vi "Test Status Correct When Collecting Case Result.vi"(8 "error in (no error)":errorcluster, 11 "Test Case In":refnum<class "Result Collector Tests.lvclass">) -> (0 "error out":errorcluster, 3 "Test Case Out":refnum<class "Result Collector Tests.lvclass">)   [LabVIEW 2020, in "Result Collector Tests.lvclass"]
uses:
  Result Collector Tests.lvclass
  C:/Program Files (x86)/National Instruments/LabVIEW 2020/vi.lib/Astemes/LUnit/Test Case.lvclass
  source/Framework/Result Collector/Result Collector.lvclass
  source/Rewrite Project/Result/Result.ctl
  source/Rewrite Project/Result/Status.ctl
  source/Rewrite Project/Result/Type.ctl
  source/Framework/Result Collector/Result Collector.lvclass/Result Collector.ctl
  <vilib>/Astemes/LUnit/Test Case.lvclass/Test Case.ctl
  7d523b10-b8d1-4baa-9334-5865d033fd32.vi
  source/Framework/Result Collector/Public/API/Collect Method Results.vi
  <vilib>/AdvancedString/Delimited String to 1D String Array.vi
  <vilib>/AdvancedString/1D String Array to Delimited String.vi
  source/Framework/Result Collector/Public/API/Collect Case Result.vi
  source/Framework/Result Collector/Public/API/Collect Suite Result.vi
  <vilib>/Astemes/LUnit/Palette/Pass.vi
  <vilib>/Astemes/LUnit/Palette/Fail.vi
  <vilib>/Astemes/LUnit/Compare Variants.vi
  <vilib>/Astemes/LUnit/Describe Comparison.vi
  <vilib>/Astemes/LUnit/Set Assertion Type.vi
  <vilib>/Astemes/LUnit/Add test result.vi
  <vilib>/Astemes/LUnit/Variant to string.vi
  <vilib>/Astemes/LUnit/LUnit Record Assertion Result.vi
  <vilib>/Astemes/LUnit/LUnit Aggregate Assertion Results.vi
  <vilib>/Astemes/LUnit/Method Result/LUnit Merge Status.vi
  <vilib>/Astemes/LUnit/LUnit Concatenate result strings.vi
  <vilib>/Utility/Data Type/Get Type Information.vi
  <vilib>/Utility/LVClass/Get LV Class Name.vi
  source/Rewrite Project/Result/Result.lvlib
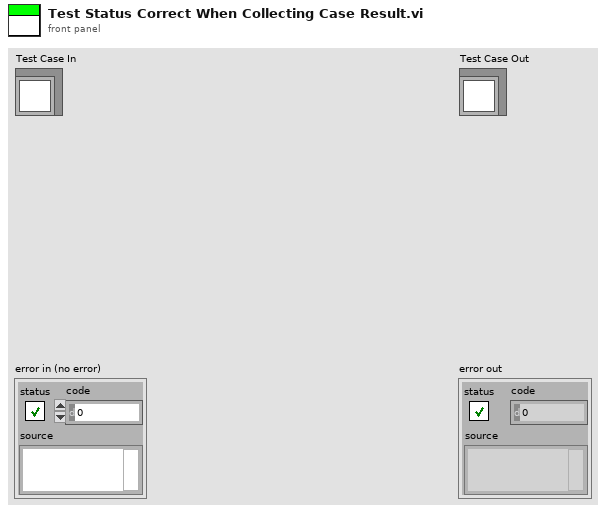
[diagram p1: front panel]
types:
  T1 = typedef "Result.lvlib/Status.ctl" = enum16{"", "Passed", "Failed", "Error", "Skipped", "Setup Error", "Broken", "Teardown Error"}
  T2 = typedef "Result.lvlib/Result.ctl" = cluster{"Name":string, "Message":string, "Description":string, "Status":T1, "Result Type":T3, "Execution Time":dbl}
  T3 = typedef "Result.lvlib/Type.ctl" = enum16{"Method", "Case", "Suite", "Pass", "Fail", "Skip", "Pass if", "Fail if", "Pass if Error", "Fail if Error", "Pass if Equal", "Fail if Equal"}
  T4 = typedef "Test Case Result.lvlib/Test Case Result.ctl" = map{string, T5}
  T5 = typedef "Method Result.lvlib/Method Result.ctl" = cluster{"Test Case":string, "Test Method Name":string, "Status":T1, "Assertion Results":T6[], "Execution time":dbl, "Result String":string}
  T6 = typedef "Assertion Result.lvlib/Assertion Result.ctl" = cluster{"Status":T1, "Message":string, "Description":string, "Assertion Type":T7}
  T7 = typedef "Result.lvlib/Assertion Type.ctl" = enum16{"None", "Pass", "Fail", "Skip", "Pass if Equal", "Fail if Equal", "Pass if Error", "Fail if Error", "Pass if", "Fail if"}
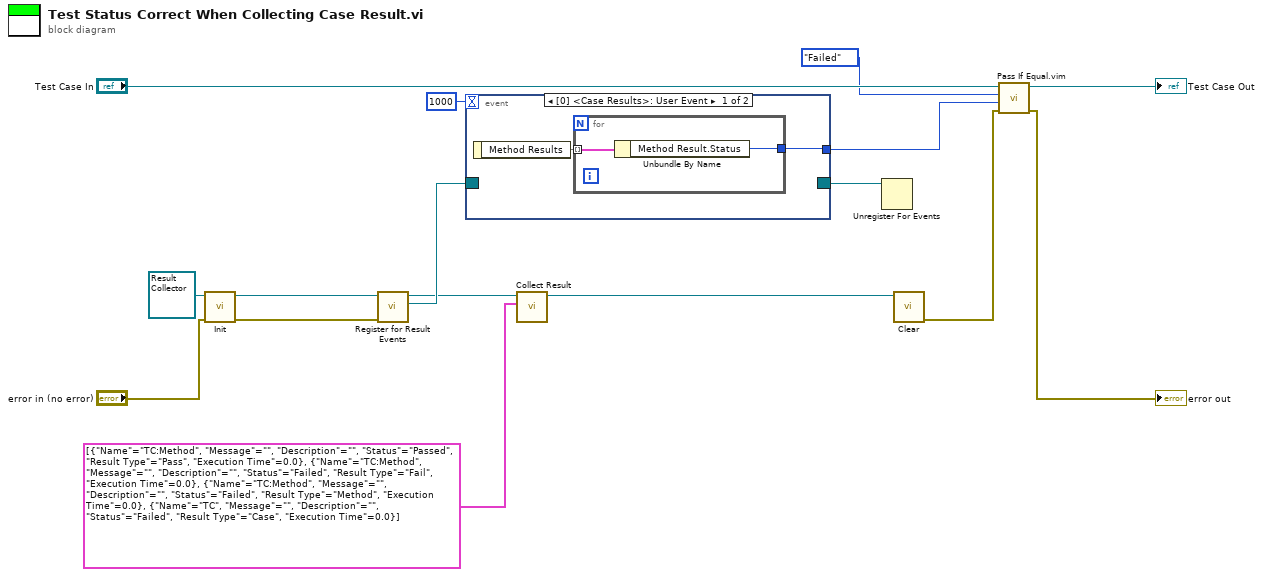
[diagram p0: block diagram]
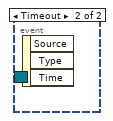
[diagram p2: hidden frame]
diagram:
  n1 = call-dynamic "Init.vi"("error in (no error)"="error in (no error)", "Report Generator In"=refnum<class "Result Collector.lvclass"> refnum) -> ("error out"=w12:errorcluster, "Report Generator Out"=w13:refnum<class "Result Collector.lvclass">)  [unwired: 8 in]
  n2 = call "Register for Result Events.vi"("error in (no error)"=w12, "Result Collector In"=w13) -> ("Event Registration Refnum"=w10:refnum<event-registration>, "Result Collector Out"=w8:refnum<class "Result Collector.lvclass">)  [unwired: 7 in, 1 out]
  n3 = event shown="[0] <Case Results>: User Event" {
    selector: w10 -> [_ _]
    dyn-events: [_ _] -> w9
    timeout: 1000 -> [_ _]
    tunnel: [w17 _] -> w5
    event User Event {
      n4 = event-data() -> ("Method Results"=w18:T4)  [unwired: 1 in]
      n5 = for {
        tunnel: w18 -> [w20] mode=indexing
        tunnel: [w19] -> w17
        n6 = Unbundle By Name(w20) -> ("Method Result.Status"=w19:T1)
      }
    }
    event Timeout {
      n7 = event-data() -> ()  [unwired: 1 in, 3 out]
    }
  }
  n8 = call "Collect Result.vi"("Results"=T2[] [{"Name"="TC:Method", "Message"="", "Description"="", "Status"=enum."Passed", "Result Type"=enum."Pass", "Execution Time"=0.0}, {"Name"="TC:Method", "Message"="", "Description"="", "Status"=enum."Failed", "Result Type"=enum."Fail", "Execution Time"=0.0}, {"Name"="TC:Method", "Message"="", "Description"="", "Status"=enum."Failed", "Result Type"=enum."Method", "Execution Time"=0.0}, {"Name"="TC", "Message"="", "Description"="", "Status"=enum."Failed", "Result Type"=enum."Case", "Execution Time"=0.0}], "Report Generator In"=w8) -> ("Report Generator Out"=w7:refnum<class "Result Collector.lvclass">)  [unwired: 9 in]
  n9 = Unregister For Events(event registration refnum=w9) -> ()  [unwired: 1 in, 1 out]
  n10 = call-dynamic "Clear.vi"("Report Generator In"=w7) -> ("error out"=w4:errorcluster)  [unwired: 9 in, 1 out]
  n11 = call "Pass If Equal.vim"("error in (no error)"=w4, "Actual"=w5, "Expected"=Status."Failed" ("Status"), "LUnit Test Case In"="Test Case In") -> ("error out"=→"error out":errorcluster, "LUnit Test Case Out"=→"Test Case Out":refnum<class "Result Collector Tests.lvclass">)  [unwired: 6 in]
